vi "Parse JSON Client Receive.vi"(8 "error in (no error)":errorcluster, 10 "JSON (UTF-8) String":string) -> (0 "error out":errorcluster, 2 "Telegram State":T1, 3 "Message":variant)   [LabVIEW 2015, in "JSON Library.lvlib"]
doc: "Created IvanLis by LabVIEW Portal\nProfile: http://labviewportal.org/memberlist.php?mode=viewprofile&u=987\neMail: IvanLisanov@gMail.com\nTelegram: https://t.me/IvanLis"
uses:
  JSON Library.lvlib
  Telegram Library/TypeDef/Telegram State.ctl
  Telegram Library/Telegram Library.lvlib
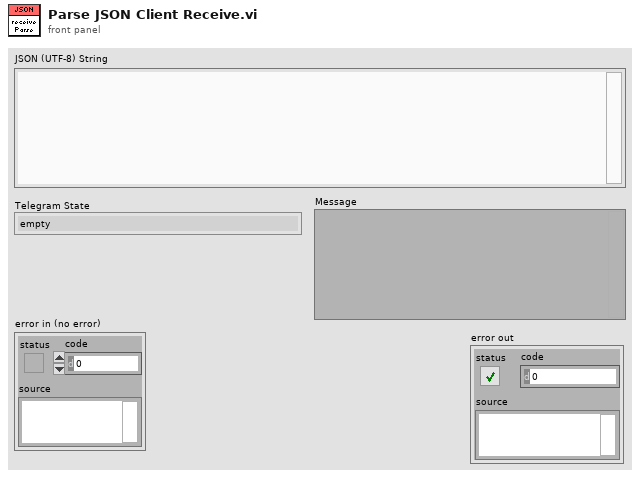
[diagram p1: front panel]
types:
  T1 = typedef "Telegram Library.lvlib/Telegram State.ctl" = enum16{"empty", "ok", "authorizationStateClosed", "authorizationStateWaitTdlibParameters", "authorizationStateWaitEncryptionKey", "authorizationStateWaitPhoneNumber", "authorizationStateWaitCode", "connectionStateWaitingForNetwork", "connectionStateConnectingToProxy", "connectionStateUpdating", "connectionStateConnecting", "connectionStateReady", "updateUser_user", "updateNewChat_chat", "updateNewMessage_Text", "updateChatLastMessage_Text", "updateDeleteMessages", "updateChatPosition", "ChatHistoryMessages_Text"}
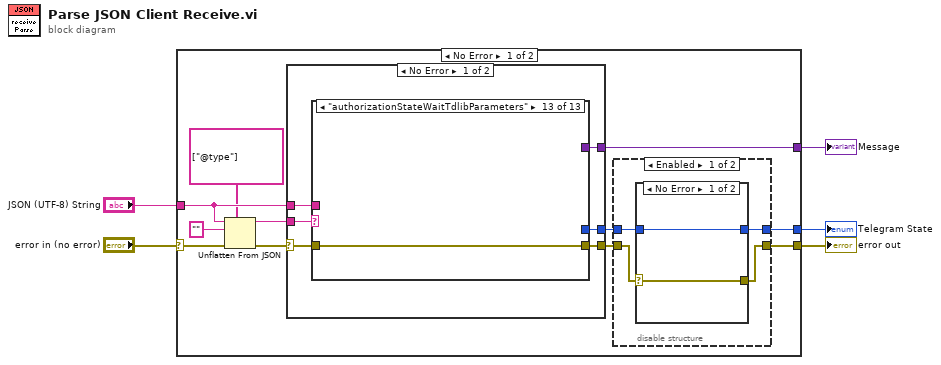
[diagram p0: block diagram]
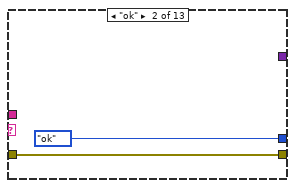
[diagram p3: hidden frame]
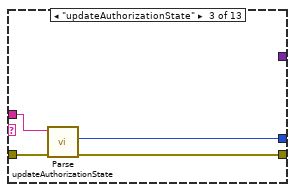
[diagram p4: hidden frame]
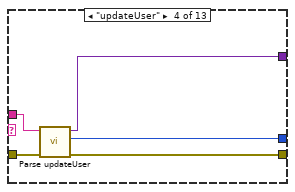
[diagram p5: hidden frame]
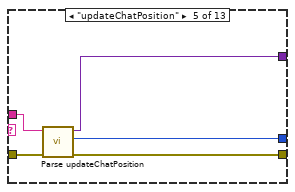
[diagram p6: hidden frame]
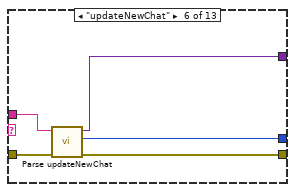
[diagram p7: hidden frame]
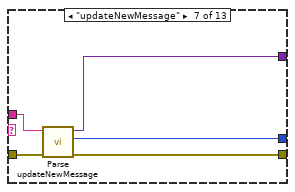
[diagram p8: hidden frame]
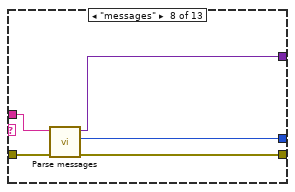
[diagram p9: hidden frame]
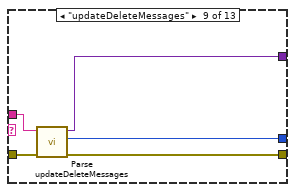
[diagram p10: hidden frame]
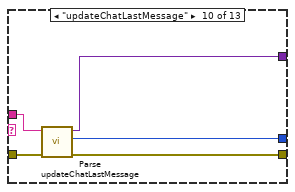
[diagram p11: hidden frame]
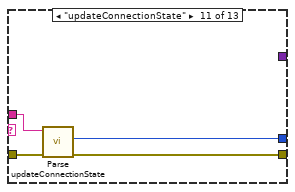
[diagram p12: hidden frame]
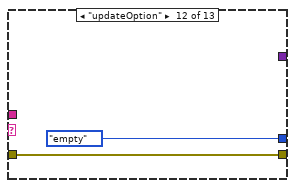
[diagram p13: hidden frame]
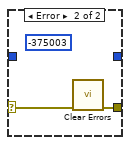
[diagram p15: hidden frame]
diagram:
  n1 = case shown="No Error" "error in (no error)" {
    selector: "error in (no error)" -> [w16 w83]
    tunnel: [w11 w83] -> w2
    tunnel: "JSON (UTF-8) String" -> [w13 _]
    tunnel: [w8 _] -> w3
    tunnel: [w12 _] -> w1
    frame No Error {
      n2 = Unflatten From JSON(path=string[] ["@type"], JSON string=w13, type and defaults="", error in (no error)=w16) -> (value=w14:string, error out=w15:errorcluster)  [unwired: 3 in]
      n3 = case shown="No Error" w15 {
        selector: w15 -> [w20 w72]
        tunnel: [w22 w72] -> w10
        tunnel: [w21 _] -> w9
        tunnel: w14 -> [w17 _]
        tunnel: w13 -> [w19 _]
        tunnel: [w18 _] -> w12
        frame No Error {
          n4 = case shown="\"authorizationStateWaitTdlibParameters\"" w17 {
            tunnel: w20 -> [w23 w24 w28 w32 w37 w42 w47 w53 w57 w62 w68 w69 w71]
            tunnel: [w23 w24 w29 w34 w39 w44 w49 w54 w59 w64 w66 w69 w71] -> w22
            tunnel: [_ Telegram_State."ok" ("Telegram State") w26 w33 w38 w43 w48 w50 w58 w63 w65 Telegram_State."empty" ("Telegram State") _] -> w21
            tunnel: w19 -> [_ _ w27 w31 w36 w41 w46 w51 w56 w60 w67 _ _]
            tunnel: [_ _ _ w30 w35 w40 w45 w52 w55 w61 _ _ _] -> w18
            frame Default {
            }
            frame "ok" {
              # "process authorization states"
            }
            frame "updateAuthorizationState" {
              # "process authorization states"
              n5 = call "Parse updateAuthorizationState.vi"("error in (no error)"=w28, "JSON (UTF-8) String"=w27) -> ("error out"=w29:errorcluster, "Telegram State"=w26:T1)  [unwired: 8 in]
            }
            frame "updateUser" {
              # "process authorization states"
              n6 = call "Parse updateUser.vi"("error in (no error)"=w32, "JSON (UTF-8) String"=w31) -> ("error out"=w34:errorcluster, "Telegram State"=w33:T1, "Variant"=w30:variant)  [unwired: 7 in]
            }
            frame "updateChatPosition" {
              # "process authorization states"
              n7 = call "Parse updateChatPosition.vi"("error in (no error)"=w37, "JSON (UTF-8) String"=w36) -> ("error out"=w39:errorcluster, "Telegram State"=w38:T1, "Variant"=w35:variant)  [unwired: 7 in]
            }
            frame "updateNewChat" {
              # "process authorization states"
              n8 = call "Parse updateNewChat.vi"("error in (no error)"=w42, "JSON (UTF-8) String"=w41) -> ("error out"=w44:errorcluster, "Telegram State"=w43:T1, "Variant"=w40:variant)  [unwired: 7 in]
            }
            frame "updateNewMessage" {
              # "process authorization states"
              n9 = call "Parse updateNewMessage.vi"("error in (no error)"=w47, "JSON (UTF-8) String"=w46) -> ("error out"=w49:errorcluster, "Telegram State"=w48:T1, "Message"=w45:variant)  [unwired: 7 in]
            }
            frame "messages" {
              # "process authorization states"
              n10 = call "Parse messages.vi"("error in (no error)"=w53, "JSON (UTF-8) String"=w51) -> ("error out"=w54:errorcluster, "Telegram State"=w50:T1, "Variant"=w52:variant)  [unwired: 7 in]
            }
            frame "updateDeleteMessages" {
              # "process authorization states"
              n11 = call "Parse updateDeleteMessages.vi"("error in (no error)"=w57, "JSON (UTF-8) String"=w56) -> ("error out"=w59:errorcluster, "Telegram State"=w58:T1, "Variant"=w55:variant)  [unwired: 7 in]
            }
            frame "updateChatLastMessage" {
              # "process authorization states"
              n12 = call "Parse updateChatLastMessage.vi"("error in (no error)"=w62, "JSON (UTF-8) String"=w60) -> ("error out"=w64:errorcluster, "Telegram State"=w63:T1, "Variant"=w61:variant)  [unwired: 7 in]
            }
            frame "updateConnectionState" {
              # "process authorization states"
              n13 = call "Parse updateConnectionState.vi"("error in (no error)"=w68, "JSON (UTF-8) String"=w67) -> ("error out"=w66:errorcluster, "Telegram State"=w65:T1)  [unwired: 8 in]
            }
            frame "updateOption" {
              # "updateOption"
            }
            frame "authorizationStateWaitTdlibParameters" {
              # "authorizationStateWaitTdlibParameters"
            }
          }
        }
        frame Error {
        }
      }
      n14 = disable-structure shown="Enabled" {
        disable-tunnel: [w76 w81] -> w11
        disable-tunnel: w10 -> [w75 w81]
        disable-tunnel: w9 -> [w74 w82]
        disable-tunnel: [w73 w82] -> w8
        frame Enabled {
          n15 = case shown="No Error" w75 {
            selector: w75 -> [w78 w79]
            tunnel: [w78 w80] -> w76
            tunnel: w74 -> [w77 _]
            tunnel: [w77 _] -> w73
            frame No Error {
            }
            frame Error {
              (unwired) -375003 ("specific error code to clear (0: all)")
              n16 = call <vilib>:"Clear Errors.vi"("error in (no error)"=w79) -> ("error out"=w80:errorcluster)  [unwired: 5 in, 1 out]
            }
          }
        }
        frame Disabled {
        }
      }
    }
    frame Error {
    }
  }
  "error out" <- w2
  "Telegram State" <- w3
  "Message" <- w1
